vi "DisableControls.vi"(0 "Operation Interface in":refnum<class "Operation Interface.lvclass">, 5 "error in (no error)":errorcluster) -> (14 "Operation Interface out":refnum<class "Operation Interface.lvclass">, 19 "error out":errorcluster)   [LabVIEW 2016, in "Operation Interface.lvclass"]
uses:
  Operation Interface.lvclass
  Operation Interface.lvclass/Operation Interface.ctl
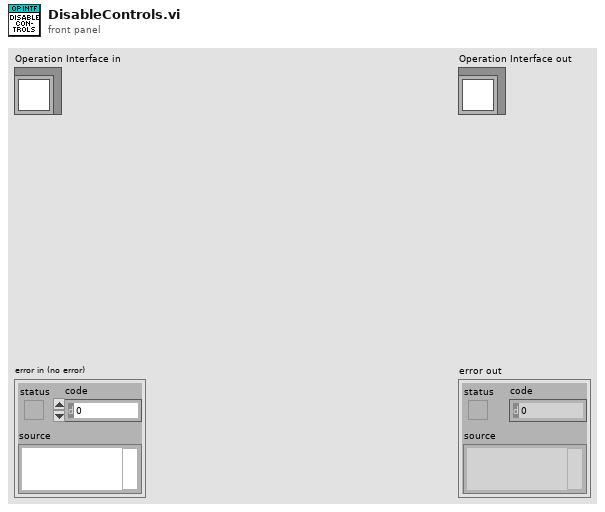
[diagram p1: front panel]
types:
  T1 = enum8{"Enabled", "Disabled", "Disabled and Grayed Out"}
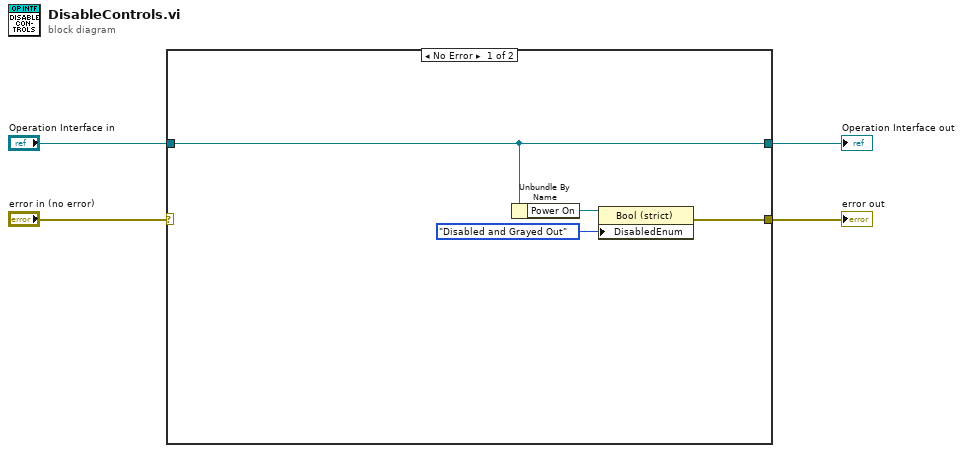
[diagram p0: block diagram]
diagram:
  n1 = case shown="No Error" "error in (no error)" {
    selector: "error in (no error)" -> [_ w10]
    tunnel: [w6 w10] -> w3
    tunnel: [w8 w9] -> w1
    tunnel: "Operation Interface in" -> [w8 w9]
    frame No Error {
      n2 = Unbundle By Name(w8) -> ("Power On"=w7:refnum<vi>)
      n3 = property class="Bool (strict)"(reference=w7, "DisabledEnum"=T1."Disabled and Grayed Out" ("Disabled")) -> (error out=w6:errorcluster)  [unwired: 1 in, 1 out]
    }
    frame Error {
    }
  }
  "error out" <- w3
  "Operation Interface out" <- w1
